vi "Create_Email_Message.vi"(10 "Responsible Mail":string, 11 "Warning":string) -> ()   [LabVIEW 2019]
uses:
  Instrument_Setup.vi
  Global/Global Variables/Data_Display_global.vi
panel:
  out "String":string
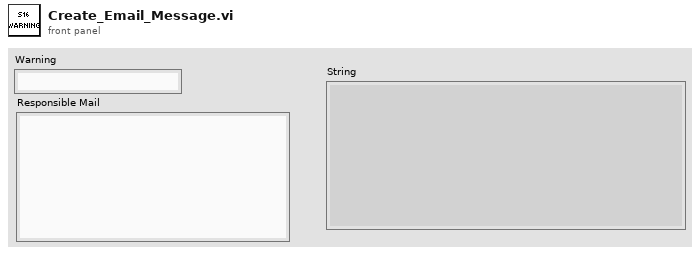
[diagram p1: front panel]
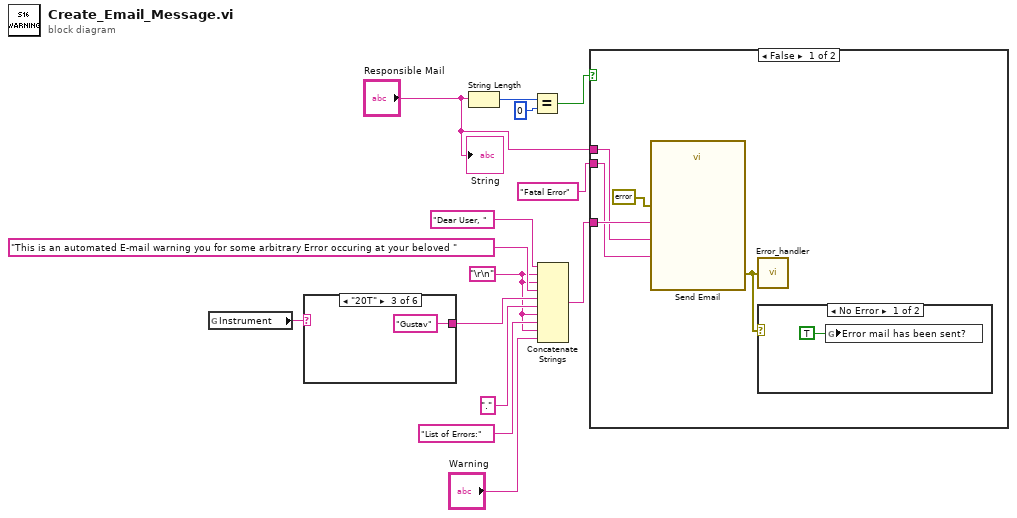
[diagram p0: block diagram]
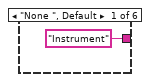
[diagram p2: hidden frame]
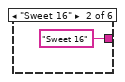
[diagram p3: hidden frame]
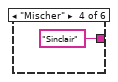
[diagram p4: hidden frame]
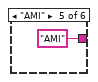
[diagram p5: hidden frame]
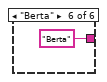
[diagram p6: hidden frame]
diagram:
  w1 = "\r\n"
  n1 = global read "Instrument_Setup.vi" "Instrument"() -> (w5:string)
  n2 = case shown="\"20T\"" w5 {
    tunnel: ["Instrument" "Sweet 16" "Gustav" "Sinclair" "AMI" "Berta"] -> w3
    frame "None ", Default {
    }
    frame "Sweet 16" {
    }
    frame "20T" {
    }
    frame "Mischer" {
    }
    frame "AMI" {
    }
    frame "Berta" {
    }
  }
  n3 = String Length(string="Responsible Mail") -> (length=w11:i32)
  n4 = Equal?(x=w11, y=0) -> (x = y?=w9:bool)
  n5 = Concatenate Strings("Dear User, ", w1, w1, "This is an automated E-mail warning you for some arbitrary Error occuring at your beloved ", w3, ".", w1, "List of Errors:", w1, "Warning") -> (w8:string)
  n6 = case shown="False" w9 {
    tunnel: w8 -> [w25 _]
    tunnel: "Responsible Mail" -> [w24 _]
    tunnel: "Fatal Error" -> [w23 _]
    frame False {
      n7 = call "Send Email"("error in"=errorcluster {"status"=FALSE, "code"=0, "source"=""} ("error constant"), "Message"=w25, "Subject"=w23, "Recipients"=w24) -> ("error out"=w21:errorcluster)  [unwired: 7 in]
      n8 = call "Error_handler.vi"("error constant"=w21) -> ()
      n9 = case shown="No Error" w21 {
        frame No Error {
          n10 = global write "Data_Display_global.vi" "Error mail has been sent?"(TRUE) -> ()
        }
        frame Error {
        }
      }
    }
    frame True {
    }
  }
  "String" <- "Responsible Mail"
